vi "ADC_SetCal.vi"(7 "DeviceIndex":u32, 8 "error in (no error)":errorcluster, 11 "CalFileName":T1) -> (0 "error out":errorcluster)   [LabVIEW 2012]
doc: "unsigned long ADC_SetCal(\nunsigned long DeviceIndex - number from 0-31 indicating to which device you wish to upload a\ncalibration file\nchar *CalFileName - either the file name of a calibration file, or a command string. A file name\ncan include the full path, or be relative to the current directory. A command string of \":AUTO:\"\ncauses this function to generate a calibration file from the calibration references and upload that.\nA command string of \":NONE:\" causes this function to generate an \"uncalibrated\" calibration file\nand upload that\n)\nThis function is currently only supported by the USB-AI16-16A and USB-AI12-16A. Lesser\nUSB analog input boards will return \"ERROR_NOT_SUPPORTED\"(equal to 50 decimal)."
uses:
  Controls/CalFileName.ctl
  Windows/System32/AIOUSB.dll
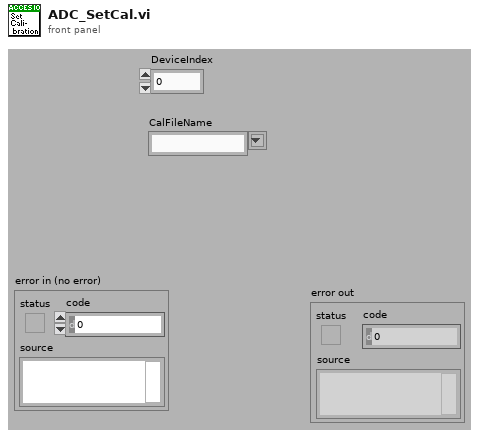
[diagram p1: front panel]
types:
  T1 = typedef "CalFileName.ctl" = string
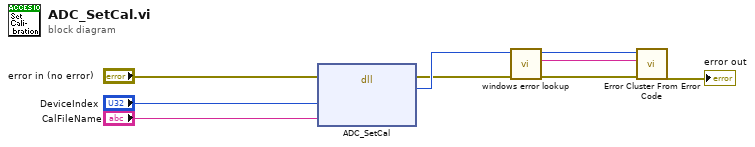
[diagram p0: block diagram]
diagram:
  n1 = dll-call lib="C:/Windows/System32/AIOUSB.dll" fn="ADC_SetCal"(error in="error in (no error)", "DeviceIndex"="DeviceIndex", "CalFileName"="CalFileName") -> (error out=w3:errorcluster, "return type"=w4:u32)  [unwired: 4 in, 1 out]
  n2 = call "windows error lookup.vi"("error in (no error)"=w3, "Error Code"=w4) -> ("error out"=w2:errorcluster, "error message (\"\")"=w5:string)  [unwired: 8 in]
  n3 = call <vilib>:"Error Cluster From Error Code.vi"("error in (no error)"=w2, "error message (\"\")"=w5, "error code (0)"=w4) -> ("error out"=→"error out":errorcluster)  [unwired: 6 in]
